vi "TcA07-004_GenericOpen.vi"(1 "Input buffer":T3="1", 3 "Invocation info":T2, 5 "error in (no error)":errorcluster, 6 "Add log to result?":bool) -> (16 "Test Data":T1 {"Numeric Measurement" format="%.2f"}, 19 "error out":errorcluster)   [LabVIEW 2020]
doc: "Test case template."
uses:
  Shared/Support_InputBuffer.ctl
  Shared/Support_InvocationInfo.ctl
  Shared/Support_TestData.ctl
  <vilib>/addons/_AddQ/G#Object/G#Object.lvclass
  TestClasses/G#SubSubClass1_class/G#SubSubClass1.lvclass
  C:/Projects/GsharpGIT/Verification/TestCases/TestClasses/G#SubClass1_class/G#SubClass1.lvclass
  TestClasses/G#SubClass1_class/G#SubClass1.lvclass
  C:/Program Files (x86)/National Instruments/LabVIEW 2020/vi.lib/addons/_AddQ/G#Object/G#Object.lvclass
panel:
  in  "Test name":string="TcA07-004 Generic Open"
  out "Test result":bool
  out "Result":string
  # "Verify that the generic open method works."
  # "Sub test case"
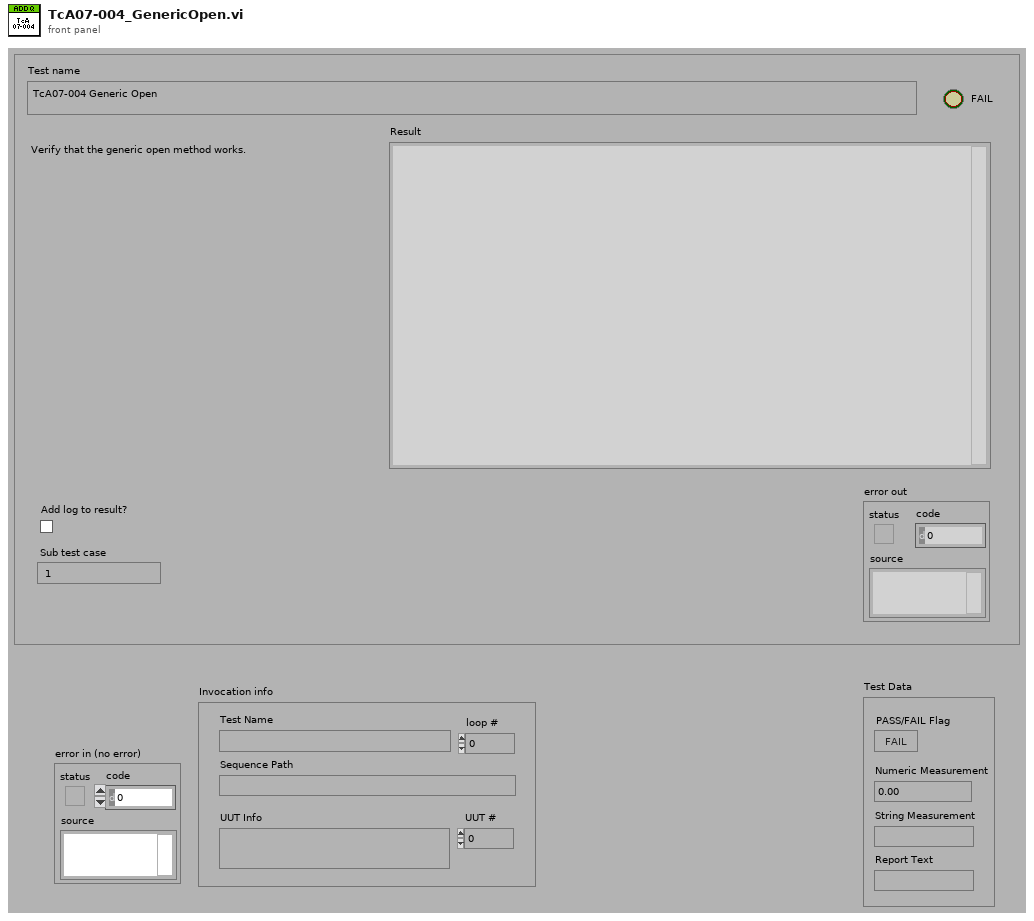
[diagram p1: front panel]
types:
  T1 = typedef "Support_TestData.ctl" = cluster{"PASS/FAIL Flag":bool, "Numeric Measurement":dbl, "String Measurement":string, "Report Text":string}
  T2 = typedef "Support_InvocationInfo.ctl" = cluster{"UUT #":i32, "loop #":i32, "UUT Info":string, "Test Name":string, "Sequence Path":path}
  T3 = typedef "Support_InputBuffer.ctl" = string
  T4 = typedef "Support_ResultType.ctl" = cluster{"Pass":bool, "Comment":string, "MeasurementValue":dbl}
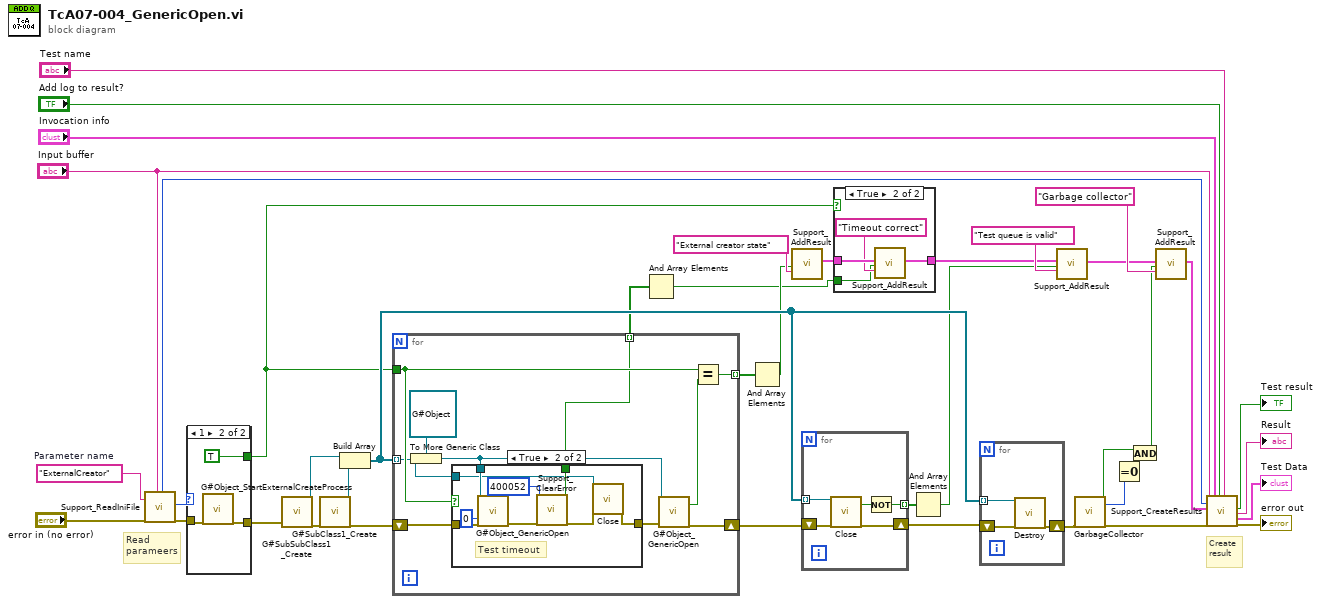
[diagram p0: block diagram]
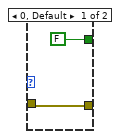
[diagram p4: hidden frame]
diagram:
  w35 = "ExternalCreator"  # Parameter name
  # "Read\nparameers"
  # "Create\nresult"
  n1 = call "Support_ReadIniFile.vi"("Parameter name"=w35, "error in (no error)"="error in (no error)", "Sub test case"="Input buffer") -> ("Timer start"=w30:u32, "Parameter1 as I32"=w21:i32, "error out"=w22:errorcluster)  [unwired: 9 in, 5 out]
  n2 = case shown="1" w21 {
    tunnel: w22 -> [w43 w46]
    tunnel: [w43 w45] -> w20
    tunnel: [FALSE TRUE] -> w1
    frame 0, Default {
    }
    frame 1 {
      n3 = call <vilib>:"G#Object_StartExternalCreateProcess.vi"("error in (no error)"=w46) -> ("error out"=w45:errorcluster)  [unwired: 18 in]
    }
  }
  n4 = call "G#SubSubClass1_Create.vi"("error in (no error)"=w20) -> ("reference out"=w18:refnum<class "G#SubSubClass1.lvclass">, "error out"=w19:errorcluster)  [unwired: 17 in]
  n5 = call "G#SubClass1_Create.vi"("error in (no error)"=w19) -> ("reference out"=w17:refnum<class "G#SubClass1.lvclass">, "error out"=w9:errorcluster)  [unwired: 16 in, 1 out]
  n6 = Build Array(w18, w17) -> (w14:refnum<class "G#SubClass1.lvclass">[])
  n7 = for {
    tunnel: w14 -> [w47] mode=indexing
    shift-right: [w55] -> w15
    shift-left: w9 -> [w51]
    tunnel: w1 -> [w49]
    tunnel: [w53] -> w7 mode=indexing
    tunnel: [w48] -> w3 mode=indexing
    n8 = To More Generic Class(target class=refnum<class "G#Object.lvclass"> refnum ("G#Object.lvclass"), reference=w47) -> (generic class reference=w50:refnum<class "G#Object.lvclass">)
    n9 = case shown="True" w49 {
      tunnel: [w57 w59] -> w52
      tunnel: w51 -> [w57 w65]
      tunnel: w50 -> [_ w64]
      tunnel: [_ w61] -> w48
      tunnel: w47 -> [_ w58]
      frame False {
      }
      frame True {
        # "Test timeout"
        n10 = call-dynamic "G#Object_GenericOpen.vi"("reference in"=w64, "timeout in ms (-1)"=0 ("timeout (ms)"), "error in (no error)"=w65) -> ("error out"=w66:errorcluster)  [unwired: 14 in, 2 out]
        n11 = call "Support_ClearError.vi"("code"=400052, "error in (no error)"=w66) -> ("Cleared?"=w61:bool, "error out"=w60:errorcluster)  [unwired: 16 in]
        n12 = call-dynamic "Close.vi"("reference in"=w58, "error in (no error)"=w60) -> ("error out"=w59:errorcluster)  [unwired: 15 in, 2 out]
      }
    }
    n13 = call-dynamic "G#Object_GenericOpen.vi"("reference in"=w50, "error in (no error)"=w52) -> ("external creator running?"=w54:bool, "error out"=w55:errorcluster)  [unwired: 15 in, 1 out]
    n14 = Equal?(x=w49, y=w54) -> (x = y?=w53:bool)
  }
  n15 = And Array Elements(Boolean array=w3) -> (logical AND=w2:bool)
  n16 = And Array Elements(Boolean array=w7) -> (logical AND=w6:bool)
  n17 = call "Support_AddResult.vi"("Pass"=w6, "Comment"="External creator state") -> ("Results out"=w5:T4[])  [unwired: 17 in]
  n18 = for {
    shift-right: [w70] -> w13
    shift-left: w15 -> [w71]
    tunnel: w14 -> [w69] mode=indexing
    tunnel: [w67] -> w12 mode=indexing
    n19 = call-dynamic "Close.vi"("reference in"=w69, "error in (no error)"=w71) -> ("not a refnum"=w68:bool, "error out"=w70:errorcluster)  [unwired: 15 in, 1 out]
    n20 = Not(x=w68) -> (.not. x?=w67:bool)
  }
  n21 = case shown="True" w1 {
    tunnel: w5 -> [w72 w76]
    tunnel: [w72 w75] -> w4
    tunnel: w2 -> [_ w73]
    frame False {
      # "Timeout\nnot used\nif external\nprocess\nnot running"
    }
    frame True {
      n22 = call "Support_AddResult.vi"("Results in"=w76, "Pass"=w73, "Comment"="Timeout correct") -> ("Results out"=w75:T4[])  [unwired: 16 in]
    }
  }
  n23 = And Array Elements(Boolean array=w12) -> (logical AND=w11:bool)
  n24 = for {
    shift-right: [w78] -> w16
    shift-left: w13 -> [w79]
    tunnel: w14 -> [w77] mode=indexing
    n25 = call-dynamic "Destroy.vi"("reference in"=w77, "error in (no error)"=w79) -> ("error out"=w78:errorcluster)  [unwired: 16 in, 1 out]
  }
  n26 = call "Support_AddResult.vi"("Results in"=w4, "Pass"=w11, "Comment"="Test queue is valid") -> ("Results out"=w10:T4[])  [unwired: 16 in]
  n27 = call <vilib>:"GarbageCollector.vi"("error in (no error)"=w16) -> ("OK"=w26:bool, "# of objects killed"=w24:i32, "error out"=w29:errorcluster)  [unwired: 16 in]
  n28 = Equal To 0?(x=w24) -> (x = 0?=w25:bool)
  n29 = And(x=w26, y=w25) -> (x .and. y?=w23:bool)
  n30 = call "Support_AddResult.vi"("Results in"=w10, "Pass"=w23, "Comment"="Garbage collector") -> ("Results out"=w28:T4[])  [unwired: 16 in]
  n31 = call "Support_CreateResults.vi"("Sub test case"="Input buffer", "Timer start"=w30, "Results"=w28, "error in (no error)"=w29, "Invocation info"="Invocation info", "Add log to result?"="Add log to result?", "Test name"="Test name") -> ("Pass/fail flag"=→"Test result":bool, "Result"=→"Result":string, "Test Data"=→"Test Data":T1, "error out"=→"error out":errorcluster)  [unwired: 9 in]
